vi "Write Interface.vi"(8 "error in (no error)":errorcluster, 10 "Interface":string, 11 "CAN_Logic in":refnum<class "CAN_Logic.lvclass">) -> (0 "error out":errorcluster, 3 "CAN_Logic out":refnum<class "CAN_Logic.lvclass">)   [LabVIEW 2021, in "CAN_Logic.lvclass"]
uses:
  CAN_Logic.lvclass
  CAN_Logic.lvclass/CAN_Logic.ctl
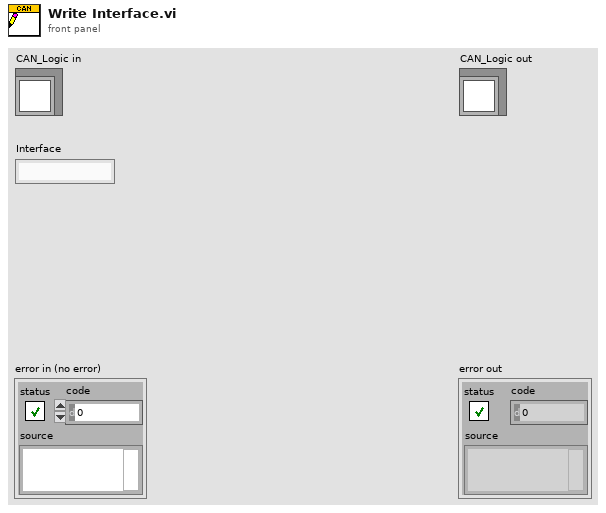
[diagram p1: front panel]
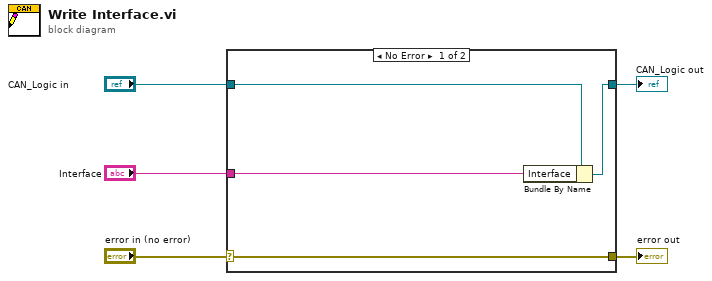
[diagram p0: block diagram]
diagram:
  n1 = case shown="No Error" "error in (no error)" {
    selector: "error in (no error)" -> [w9 w10]
    tunnel: [w9 w10] -> w4
    tunnel: [w7 w11] -> w2
    tunnel: "CAN_Logic in" -> [w8 w11]
    tunnel: "Interface" -> [w6 _]
    frame No Error {
      n2 = Bundle By Name(cluster=w8, "Interface"=w6) -> (w7:refnum<class "CAN_Logic.lvclass">)
    }
    frame Error {
    }
  }
  "error out" <- w4
  "CAN_Logic out" <- w2
